vi "Disabled - Const Array to Output (SubVI).vi"(2 "Constant cluster":T1, 4 "Constants Numeric Array":dbl[](array[numeric])) -> (0 "Constant cluster output":T1 {"15. Center-Center Sector Distance" format="%_6f"; "14. Inches / Tick Drivetrain" format="%_6f"; "13. Auton I Output Limit Drive Straight Gain" format="%_6f"; "12. Auton Deriv Drive Straight Gain" format="%_6f"; "11. Auton Int Drive Straight Gain" format="%_6f"; "10. Auton Prop Drive Straight Gain" format="%_6f"; "9. Auton I Output Limit Turn Gain" format="%_6f"; "8. Auton Deriv Turn Gain" format="%_6f"; "7. Auton Int Turn Gain" format="%_6f"; "1. Auton Prop Drive Gain" format="%_6f"; "2. Auton Int Drive Gain" format="%_6f"; "3. Auton Deriv Drive Gain" format="%_6f"; "4. I Output Drive  Limit" format="%_6f"; "5. Auto Drive Cheat (%)" format="%_6f"; "6. Auton Prop Turn Gain" format="%_6f"})   [LabVIEW 2019]
doc: "Load Numeric Array into Named Cluster so they can be unbundled by name and used."
uses:
  Disabled - Constant Cluster Typedef.ctl
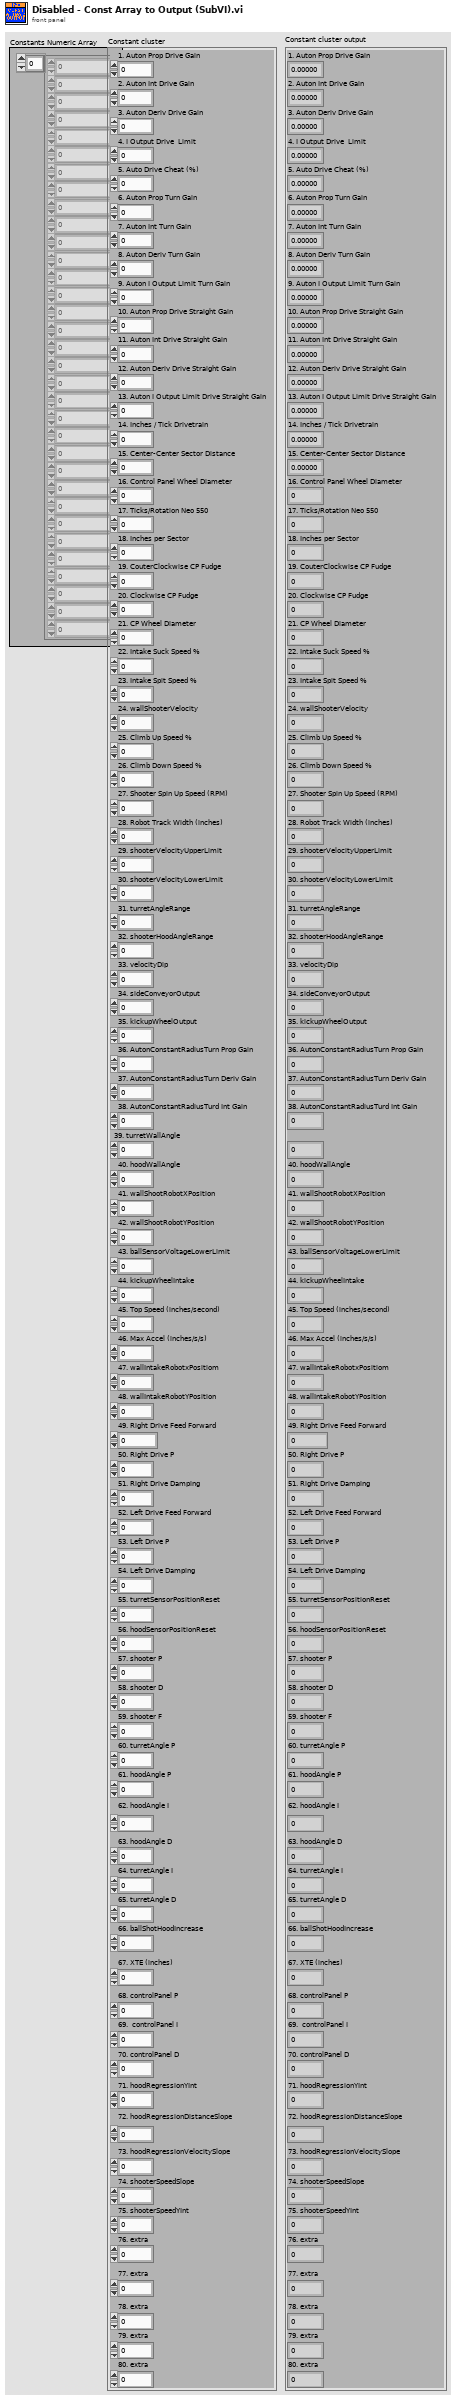
[diagram p1: front panel]
types:
  T1 = typedef "Disabled - Constant Cluster Typedef.ctl" = cluster{"1. Auton Prop Drive Gain":dbl, "2. Auton Int Drive Gain":dbl, "3. Auton Deriv Drive Gain":dbl, "4. I Output Drive  Limit":dbl, "5. Auto Drive Cheat (%)":dbl, "6. Auton Prop Turn Gain":dbl, "7. Auton Int Turn Gain":dbl, "8. Auton Deriv Turn Gain":dbl, "9. Auton I Output Limit Turn Gain":dbl, "10. Auton Prop Drive Straight Gain":dbl, "11. Auton Int Drive Straight Gain":dbl, "12. Auton Deriv Drive Straight Gain":dbl, "13. Auton I Output Limit Drive Straight Gain":dbl, "14. Inches / Tick Drivetrain":dbl, "15. Center-Center Sector Distance":dbl, "16. Control Panel Wheel Diameter":dbl, "17. Ticks/Rotation Neo 550":dbl, "18. Inches per Sector":dbl, "19. CouterClockwise CP Fudge":dbl, "20. Clockwise CP Fudge":dbl, "21. CP Wheel Diameter":dbl, "22. Intake Suck Speed %":dbl, "23. Intake Spit Speed %":dbl, "24. wallShooterVelocity":dbl, "25. Climb Up Speed %":dbl, "26. Climb Down Speed %":dbl, "27. Shooter Spin Up Speed (RPM)":dbl, "28. Robot Track Width (inches)":dbl, "29. shooterVelocityUpperLimit":dbl, "30. shooterVelocityLowerLimit":dbl, "31. turretAngleRange":dbl, "32. shooterHoodAngleRange":dbl, "33. velocityDip":dbl, "34. sideConveyorOutput":dbl, "35. kickupWheelOutput":dbl, "36. AutonConstantRadiusTurn Prop Gain":dbl, "37. AutonConstantRadiusTurn Deriv Gain":dbl, "38. AutonConstantRadiusTurd Int Gain":dbl, "39. turretWallAngle":dbl, "40. hoodWallAngle":dbl, "41. wallShootRobotXPosition":dbl, "42. wallShootRobotYPosition":dbl, "43. ballSensorVoltageLowerLimit":dbl, "44. kickupWheelIntake":dbl, "45. Top Speed (inches/second)":dbl, "46. Max Accel (inches/s/s)":dbl, "47. wallIntakeRobotxPositiom":dbl, "48. wallIntakeRobotYPosition":dbl, "49. Right Drive Feed Forward":dbl, "50. Right Drive P":dbl, "51. Right Drive Damping":dbl, "52. Left Drive Feed Forward":dbl, "53. Left Drive P":dbl, "54. Left Drive Damping":dbl, "55. turretSensorPositionReset":dbl, "56. hoodSensorPositionReset":dbl, "57. shooter P":dbl, "58. shooter D":dbl, "59. shooter F":dbl, "60. turretAngle P":dbl, "61. hoodAngle P":dbl, "62. hoodAngle I":dbl, "63. hoodAngle D":dbl, "64. turretAngle I":dbl, "65. turretAngle D":dbl, "66. ballShotHoodIncrease":dbl, "67. XTE (inches)":dbl, "68. controlPanel P":dbl, "69.  controlPanel I":dbl, "70. controlPanel D":dbl, "71. hoodRegressionYInt":dbl, "72. hoodRegressionDistanceSlope":dbl, "73. hoodRegressionVelocitySlope":dbl, "74. shooterSpeedSlope":dbl, "75. shooterSpeedYInt":dbl, "76. extra":dbl, "77. extra":dbl, "78. extra":dbl, "79. extra":dbl, "80. extra":dbl}
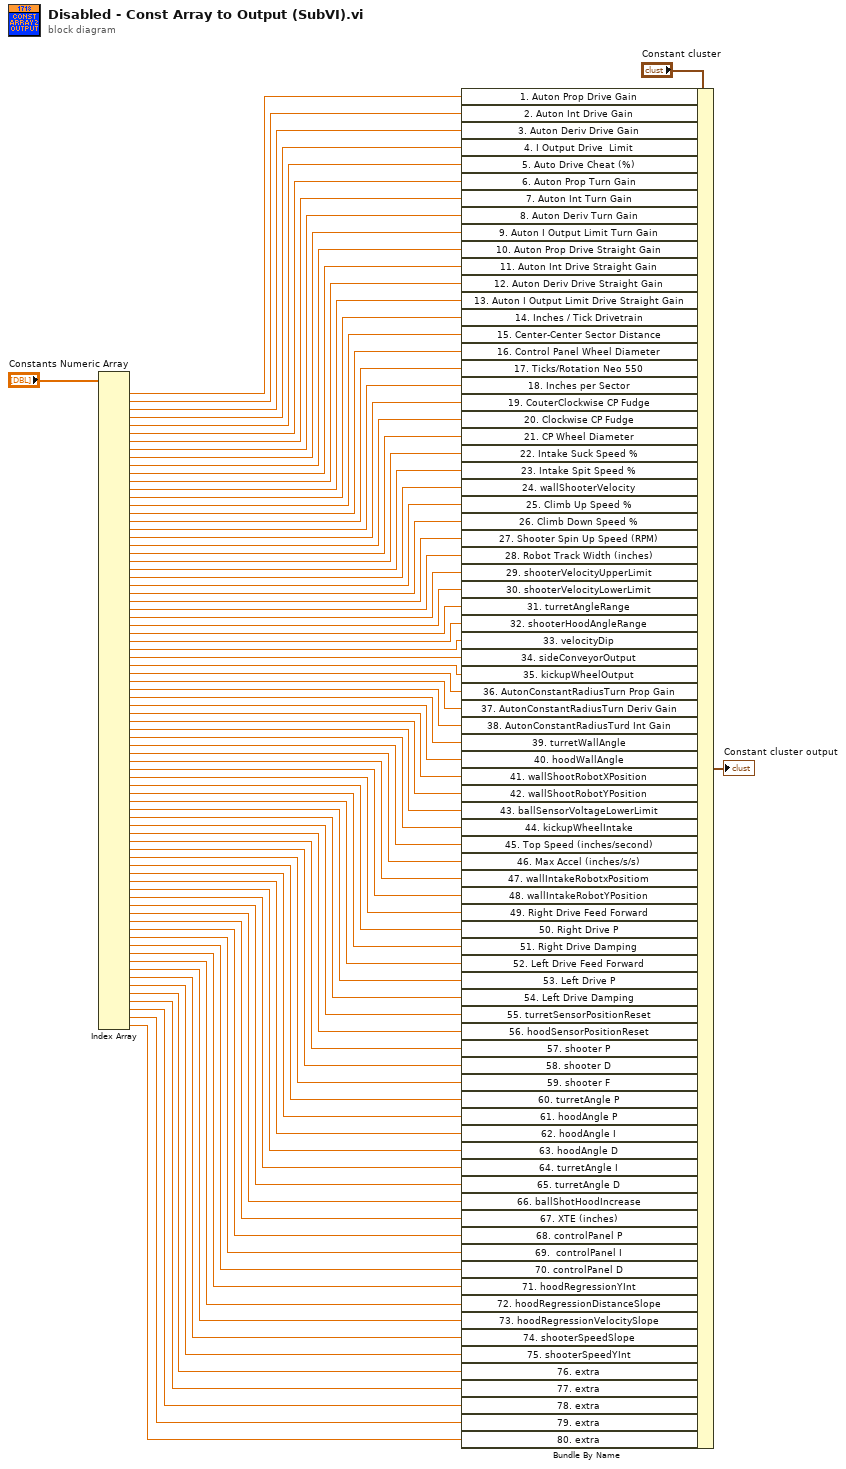
[diagram p0: block diagram]
diagram:
  n1 = Index Array(array="Constants Numeric Array") -> (element #1=w83:dbl, element #2=w82:dbl, element #3=w81:dbl, element #4=w72:dbl, element #5=w71:dbl, element #6=w70:dbl, element #7=w79:dbl, element #8=w78:dbl, element #9=w77:dbl, element #10=w76:dbl, element #11=w75:dbl, element #12=w74:dbl, element #13=w73:dbl, element #14=w69:dbl, element #15=w68:dbl, element #16=w66:dbl, element #17=w67:dbl, element #18=w65:dbl, element #19=w64:dbl, element #20=w63:dbl, element #21=w55:dbl, element #22=w62:dbl, element #23=w61:dbl, element #24=w60:dbl, element #25=w59:dbl, element #26=w58:dbl, element #27=w57:dbl, element #28=w56:dbl, element #29=w53:dbl, element #30=w52:dbl, element #31=w50:dbl, element #32=w51:dbl, element #33=w48:dbl, element #34=w47:dbl, element #35=w46:dbl, element #36=w45:dbl, element #37=w44:dbl, element #38=w43:dbl, element #39=w42:dbl, element #40=w41:dbl, element #41=w40:dbl, element #42=w39:dbl, element #43=w38:dbl, element #44=w37:dbl, element #45=w36:dbl, element #46=w35:dbl, element #47=w34:dbl, element #48=w33:dbl, element #49=w32:dbl, element #50=w31:dbl, element #51=w30:dbl, element #52=w29:dbl, element #53=w28:dbl, element #54=w27:dbl, element #55=w26:dbl, element #56=w25:dbl, element #57=w24:dbl, element #58=w23:dbl, element #59=w22:dbl, element #60=w21:dbl, element #61=w20:dbl, element #62=w19:dbl, element #63=w18:dbl, element #64=w17:dbl, element #65=w16:dbl, element #66=w15:dbl, element #67=w14:dbl, element #68=w13:dbl, element #69=w12:dbl, element #70=w11:dbl, element #71=w10:dbl, element #72=w9:dbl, element #73=w8:dbl, element #74=w7:dbl, element #75=w6:dbl, element #76=w5:dbl, element #77=w4:dbl, element #78=w3:dbl, element #79=w2:dbl, element #80=w1:dbl)  [unwired: 80 in]
  n2 = Bundle By Name(cluster="Constant cluster", "1. Auton Prop Drive Gain"=w83, "2. Auton Int Drive Gain"=w82, "3. Auton Deriv Drive Gain"=w81, "4. I Output Drive  Limit"=w72, "5. Auto Drive Cheat (%)"=w71, "6. Auton Prop Turn Gain"=w70, "7. Auton Int Turn Gain"=w79, "8. Auton Deriv Turn Gain"=w78, "9. Auton I Output Limit Turn Gain"=w77, "10. Auton Prop Drive Straight Gain"=w76, "11. Auton Int Drive Straight Gain"=w75, "12. Auton Deriv Drive Straight Gain"=w74, "13. Auton I Output Limit Drive Straight Gain"=w73, "14. Inches / Tick Drivetrain"=w69, "15. Center-Center Sector Distance"=w68, "16. Control Panel Wheel Diameter"=w66, "17. Ticks/Rotation Neo 550"=w67, "18. Inches per Sector"=w65, "19. CouterClockwise CP Fudge"=w64, "20. Clockwise CP Fudge"=w63, "21. CP Wheel Diameter"=w55, "22. Intake Suck Speed %"=w62, "23. Intake Spit Speed %"=w61, "24. wallShooterVelocity"=w60, "25. Climb Up Speed %"=w59, "26. Climb Down Speed %"=w58, "27. Shooter Spin Up Speed (RPM)"=w57, "28. Robot Track Width (inches)"=w56, "29. shooterVelocityUpperLimit"=w53, "30. shooterVelocityLowerLimit"=w52, "31. turretAngleRange"=w50, "32. shooterHoodAngleRange"=w51, "33. velocityDip"=w48, "34. sideConveyorOutput"=w47, "35. kickupWheelOutput"=w46, "36. AutonConstantRadiusTurn Prop Gain"=w45, "37. AutonConstantRadiusTurn Deriv Gain"=w44, "38. AutonConstantRadiusTurd Int Gain"=w43, "39. turretWallAngle"=w42, "40. hoodWallAngle"=w41, "41. wallShootRobotXPosition"=w40, "42. wallShootRobotYPosition"=w39, "43. ballSensorVoltageLowerLimit"=w38, "44. kickupWheelIntake"=w37, "45. Top Speed (inches/second)"=w36, "46. Max Accel (inches/s/s)"=w35, "47. wallIntakeRobotxPositiom"=w34, "48. wallIntakeRobotYPosition"=w33, "49. Right Drive Feed Forward"=w32, "50. Right Drive P"=w31, "51. Right Drive Damping"=w30, "52. Left Drive Feed Forward"=w29, "53. Left Drive P"=w28, "54. Left Drive Damping"=w27, "55. turretSensorPositionReset"=w26, "56. hoodSensorPositionReset"=w25, "57. shooter P"=w24, "58. shooter D"=w23, "59. shooter F"=w22, "60. turretAngle P"=w21, "61. hoodAngle P"=w20, "62. hoodAngle I"=w19, "63. hoodAngle D"=w18, "64. turretAngle I"=w17, "65. turretAngle D"=w16, "66. ballShotHoodIncrease"=w15, "67. XTE (inches)"=w14, "68. controlPanel P"=w13, "69.  controlPanel I"=w12, "70. controlPanel D"=w11, "71. hoodRegressionYInt"=w10, "72. hoodRegressionDistanceSlope"=w9, "73. hoodRegressionVelocitySlope"=w8, "74. shooterSpeedSlope"=w7, "75. shooterSpeedYInt"=w6, "76. extra"=w5, "77. extra"=w4, "78. extra"=w3, "79. extra"=w2, "80. extra"=w1) -> (→"Constant cluster output":T1)
